vi "Define Parameter.vi"(8 "error in (no error)":errorcluster, 11 "Analyze BeamDeviation in":refnum<class "Analyze BeamDeviation.lvclass">) -> (0 "error out":errorcluster, 3 "Analyze BeamDeviation out":refnum<class "Analyze BeamDeviation.lvclass">)   [LabVIEW 2020, in "Analyze.lvlib" / "Analyze BeamDeviation.lvclass"]
uses:
  Analyze BeamDeviation.lvclass
  Analyze Parameter/Analyze Parameter Target Point/Target Point.lvclass
  C:/POLARIS Programme/POLARIS-AS-3-Cams/Submodules/HIJ Vision/Analyze/Analyze Parameter/Analyze Parameter Base/Analyze Parameter Base.lvclass
  Analyze BaseClass/Analyze BaseClass/Analyze BaseClass.lvclass
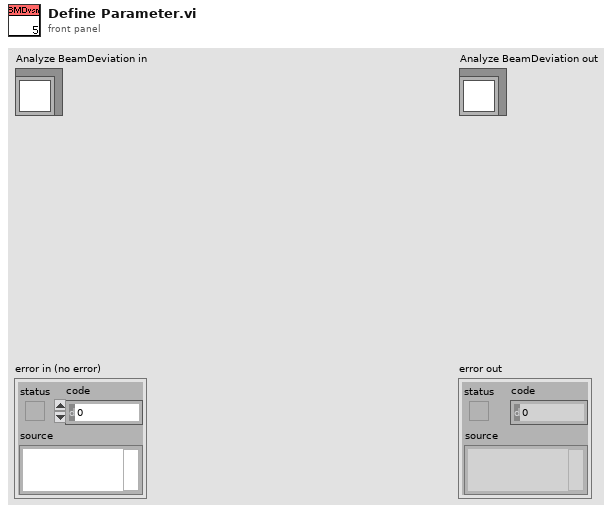
[diagram p1: front panel]
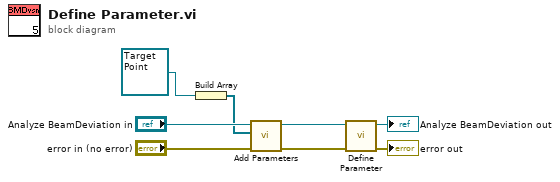
[diagram p0: block diagram]
diagram:
  n1 = Build Array(refnum<class "Target Point.lvclass"> refnum ("Target Point")) -> (w2:refnum<class "Target Point.lvclass">[])
  n2 = call-dynamic "Add Parameters.vi"("error in (no error)"="error in (no error)", "Parameters"=w2, "Analyze BaseClass in"="Analyze BeamDeviation in") -> ("error out"=w4:errorcluster, "Analyze BaseClass out"=w5:refnum<class "Analyze BeamDeviation.lvclass">)  [unwired: 7 in]
  n3 = call-parent "Define Parameter.vi"("error in (no error)"=w4, "Analyze BaseClass in"=w5) -> ("error out"=→"error out":errorcluster, "Analyze BaseClass out"=→"Analyze BeamDeviation out":refnum<class "Analyze BeamDeviation.lvclass">)  [unwired: 8 in]
